vi "CheckResultMatchRes.vi"(8 "Your Suppose":i64[][](array[numeric]), 11 "Last Draw":i64[](array[numeric])) -> (0 "Matches array":i64[][](array[numeric]), 1 "Matches":i32[](array[numeric]), 2 "Your Suppose":i64[][](array[numeric]), 3 "Last Draw":i64[](array[numeric]))   [LabVIEW 2023]
panel:
  out "YSuppSize":i32
  out "Matches":i32[](array[numeric])
  out "Your Suppose":i32[][](array[numeric])
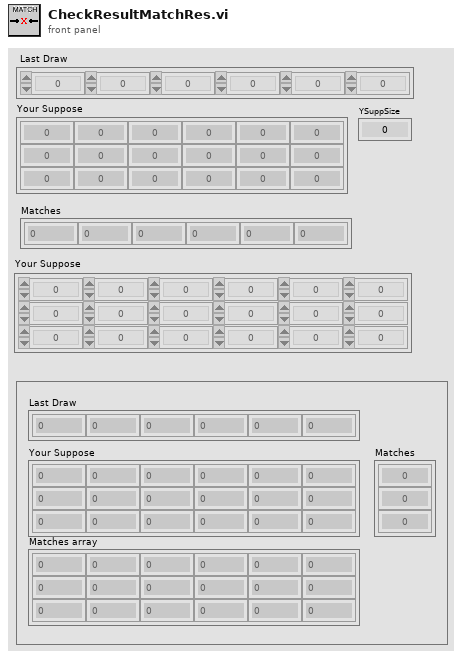
[diagram p1: front panel]
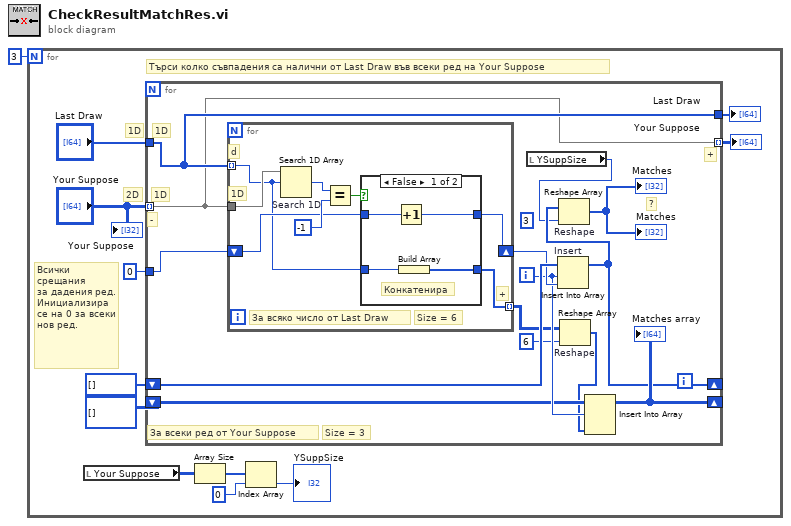
[diagram p0: block diagram]
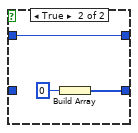
[diagram p2: hidden frame]
diagram:
  n1 = for {
    N: 3 -> [_]
    # "Всички срещания\nза дадения ред. Инициализира се на 0 за всеки нов ред."
    # "Търси колко съвпадения са налични от Last Draw във всеки ред на Your Suppose"
    # "2D"
    # "1D"
    n2 = local read "Your Suppose"() -> (w5:i32[][])
    n3 = for {
      tunnel: "Your Suppose" -> [w22] mode=indexing
      tunnel: "Last Draw" -> [w23]
      shift-right: [w14] -> _
      shift-left: i32[] [] -> [w26]
      tunnel: 0 -> [w24]
      tunnel: [w23] -> w8
      tunnel: [w22] -> w7 mode=indexing
      shift-right: [w18] -> _
      shift-left: i64[][] [] -> [w19]
      i -> [w20]
      (unwired) 3 ("dimension size")
      # "?"
      # "Size = 3"
      # "За всеки ред от Your Suppose"
      # "-"
      # "+"
      # "1D"
      # "1D"
      n4 = for {
        tunnel: w22 -> [w34]
        tunnel: w23 -> [w28] mode=indexing
        shift-right: [w30] -> w25
        shift-left: w24 -> [w29]
        tunnel: [w27] -> w17 mode=indexing
        # "Size = 6"
        # "За всяко число от Last Draw"
        # "+"
        # "1D"
        # "d"
        n5 = Search 1D Array "Search 1D"(1D array=w34, element=w28) -> (index of element=w33:i32)  [unwired: 1 in]
        n6 = Equal?(x=w33, y=-1) -> (x = y?=w31:bool)
        n7 = case shown="False" w31 {
          tunnel: [w38 w41] -> w30
          tunnel: w29 -> [w37 w41]
          tunnel: w28 -> [w36 _]
          tunnel: [w35 w40] -> w27
          frame False {
            # "Конкатенира"
            n8 = Increment(x=w37) -> (x+1=w38:i32)
            n9 = Build Array "Build Array"(w36) -> (w35:i64[])
          }
          frame True {
            n10 = Build Array "Build Array"(i64 0 ("element")) -> (w40:i64[])
          }
        }
      }
      n11 = local read "YSuppSize"() -> (w13:i32)
      n12 = Insert Into Array "Insert"(array=w26, index=w20, new element=w25) -> (w14:i32[])
      n13 = Reshape Array "Reshape"(w14, w13) -> (→"Matches" →"Matches":i32[])
      n14 = Reshape Array "Reshape"(w17, 6 ("dimension size")) -> (w15:i64[])
      n15 = Insert Into Array "Insert Into Array"(array=w19, index (row)=w20, new element=w15) -> (w18:i64[][])  [unwired: 1 in]
      "Matches array" <- w18
    }
    "Last Draw" <- w8
    "Your Suppose" <- w7
    n16 = Array Size(array=w5) -> (size(s)=w4:i32[])
    n17 = Index Array(array=w4, index=0) -> (element=→"YSuppSize":i32)
    "Your Suppose" <- "Your Suppose"
  }
